vi "Funktionen Schalten NEU.vi"(8 "Fehler (Eingang)":errorcluster) -> (0 "Fehler (Ausgang)":errorcluster, 2 "Zustand":T1)   [LabVIEW 2020, in "Allgemein.lvlib"]
uses:
  Allgemein.lvlib
  Aktionen FGV Dichtheitstest.ctl
  Verwaltung/Verwaltung - cRIO.lvlib
  Verwaltung/FGV OUT Aktionen.ctl
  Regler/Regler.lvlib
  Regler/FGV Daten Regler Aktionen.ctl
  FGV Analysator aktiv.ctl
  Anlage Spuelen Aktionen.ctl
  FGV Zustaende Aktionen.ctl
  Aktion FGV Klima.ctl
  Funktionstasten/Zustaende.ctl
  Funktionstasten/Funktionstasten.lvlib
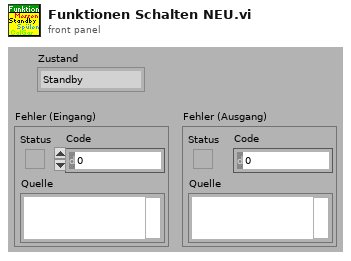
[diagram p1: front panel]
types:
  T1 = typedef "Funktionstasten.lvlib/Zustaende.ctl" = enum16{"Standby", "Pause", "Eco", "Messen", "Kalibrieren", "Spülen Filter", "Spülen Leitung", "Umgebungsluft", "0-Gas", "Cal-Gas", "CG zu PNS", "-------------", "Init 1", "Init 2", "Init 3", "Init 4", "Messen vorbereiten", "Messen durchführen", "Exit"}
  T2 = typedef "Allgemein.lvlib/Aktionen FGV Dichtheitstest.ctl" = enum16{"lesen", "schreiben"}
  T3 = typedef "Allgemein.lvlib/FGV Zustaende Aktionen.ctl" = enum16{"lesen", "Zustand PC", "Zustand cRIO", "Bildnummer", "Samplepoint", "Sysloglevel"}
  T4 = enum16{"Standby", "Pause", "Eco", "Messen", "Kalibrieren", "Spülen Filter", "Spülen Leitung", "Umgebungsluft", "0-Gas", "Cal-Gas 1", "CG zu PNS", "-------------", "Init 1", "Init 2", "Init 3", "Init 4", "Messen vorbereiten", "Messen durchführen", "Exit"}
  T5 = typedef "Regler.lvlib/FGV Daten Regler Aktionen.ctl" = enum16{"lesen", "Out%", "Heizung EIN"}
  T6 = typedef "Verwaltung - cRIO.lvlib/FGV OUT Aktionen.ctl" = enum16{"lesen", "ANA OUT", "DO 0-31", "DO 32-47"}
  T7 = typedef "Allgemein.lvlib/Anlage Spuelen Aktionen.ctl" = enum16{"lesen", "spülen?"}
  T8 = typedef "Allgemein.lvlib/FGV Analysator aktiv.ctl" = enum16{"lesen", "Analysator", "CG Aufschaltung", "KAL Zustand", "AutaKal GT?"}
  T9 = typedef "Allgemein.lvlib/Aktion FGV Klima.ctl" = enum16{"lesen", "Klimaanlage", "Container", "PNS"}
  T10 = typedef "EPA 1065.lvlib/Dichtheitstest 1065-345.lvlib/Aktion Leak check durchfuehren.ctl" = enum16{"initialisieren", "Unterdruck erzeugen", "Ventile schließen", "Warten", "Auswertung", "fertig", "PDF erstellen"}
  T11 = typedef "Erweiterte Konfig.lvlib/Aktionen Dichtheitstest.ctl" = enum16{"Initialisieren", "Unterdruck aufbauen", "Prop schließen", "Warten", "Auswertung", "Fertig"}
  T12 = cluster{"-20Y2":bool, "-20Y7":bool, "-21Y5":bool, "-22Y4":bool, "Absaugung":bool}
  T13 = typedef "Status Analysatoren.lvlib/Status Analysatoren_Anzeige.ctl" = cluster{"FT-IR":bool, "FID":bool, "PMA":bool}
  T14 = cluster{"20Y5":bool, "20Y6":bool, "20Y7":bool, "20Y8":bool, "21Y3":bool, "22Y3":bool, "23Y1":bool, "23Y2":bool, "23Y3":bool, "23Y4":bool, "27Y2":bool, "27Y3":bool, "27Y4":bool, "Absaugung":bool, "Kondensatpumpe":bool, "21Y5":bool}
  T15 = cluster{"-23Y1 (CG1)":bool, "-23Y2 (CG2)":bool, "-23Y3 (CG3-10)":bool, "-23Y4 (N2)":bool, "-23Y5":bool, "-27Y2":bool, "-20Y5":bool, "-20Y6":bool, "-20Y7":bool, "-20Y8":bool, "-27Y3":bool, "-27Y4":bool, "Pumpe":bool, "Kondensat":bool, "-22Y3":bool, "-20Y2":bool, "-21Y3":bool, "Absaugung":bool, "-21Y5":bool, "CG zu Entnahme":bool, "-20Y2 (CG3)":bool, "-20Y3 (CG4)":bool, "-20Y4 (CG5)":bool, "-20Y5 (CG6)":bool, "-20Y6 (CG7)":bool, "-20Y7 (CG8)":bool, "-20Y8 (CG9)":bool, "-21Y1 (CG10)":bool}
  T16 = typedef "Verwaltung - cRIO.lvlib/Digital Ausgaenge 32-63.ctl" = cluster{"O32: Messgaspumpe EIN":bool, "O33: (Umgebungsluftpumpe)":bool, "O34: (Kondensatpumpe GK)":bool, "O35: Klima/Lüfter EIN":bool, "O36: Versorgung Heizungen":bool, "O37: Versorgung Heizungen":bool, "O38: (Gaskühler EIN (Freigabe))":bool, "O39: Störung FAS LP":bool, "O40: (Heizung Filterblock)":bool, "O41: Heizung HL zu FT-IR":bool, "O42: Heizung HL Extern SP1":bool, "O43: Heizung HL Extern SP2":bool, "O44: Heizung Reserve":bool, "O45: Heizung Reserve":bool, "O46: Statusbeleuchtung grün":bool, "O47: Statusbeleuchtung rot":bool}
  T17 = typedef "Verwaltung - cRIO.lvlib/Digital Ausgaenge 0-31.ctl" = cluster{"O0: Druckluft Versorgung":bool, "O1: CG 3 (FB Eingang 1)":bool, "O2: CG 4 (Kühlung FT-IR EIN)":bool, "O3: CG 5 (FB Bypass)":bool, "O4: CG 6 (FB CalGas)":bool, "O5: CG 7 (FB spülen/UL)":bool, "O6: CG 8 (FB zum FT-IR)":bool, "O7: CG 9 (FB zum FID)":bool, "O8: CG 10 (FB Reserve)":bool, "O9: (FB Reserve)":bool, "O10: (FB Umgebungsluft FID)":bool, "O11: (FB zum Gaskühler)":bool, "O12: FB Stickstoff zu FT-IR":bool, "O13: (FB Druckluft/UL)":bool, "O14: (Purifier deaktivieren)":bool, "O15: (Umschaltung Purifier/Stickstoff)":bool, "O16: N2 Einblasung":bool, "O17: LSP LN2 Nachfüllung":bool, "O18: (Reserve)":bool, "O19: (Pumpe Eingang1)":bool, "O20: (Pumpe Eingang2)":bool, "O21: (Pumpe Spülen1)":bool, "O22: (Pumpe Spülen2)":bool, "O23: (Reserve)":bool, "O24: CalGas 1":bool, "O25: CalGas 2":bool, "O26: CG 3-10 (CalGas 3)":bool, "O27: Stickstoff aufschalten":bool, "O28: CG zu PNS":bool, "O29: FTIR Standby Spülung":bool, "O30: CG zu Entnahme(T90)":bool, "O31: (Purifier regenerieren)":bool}
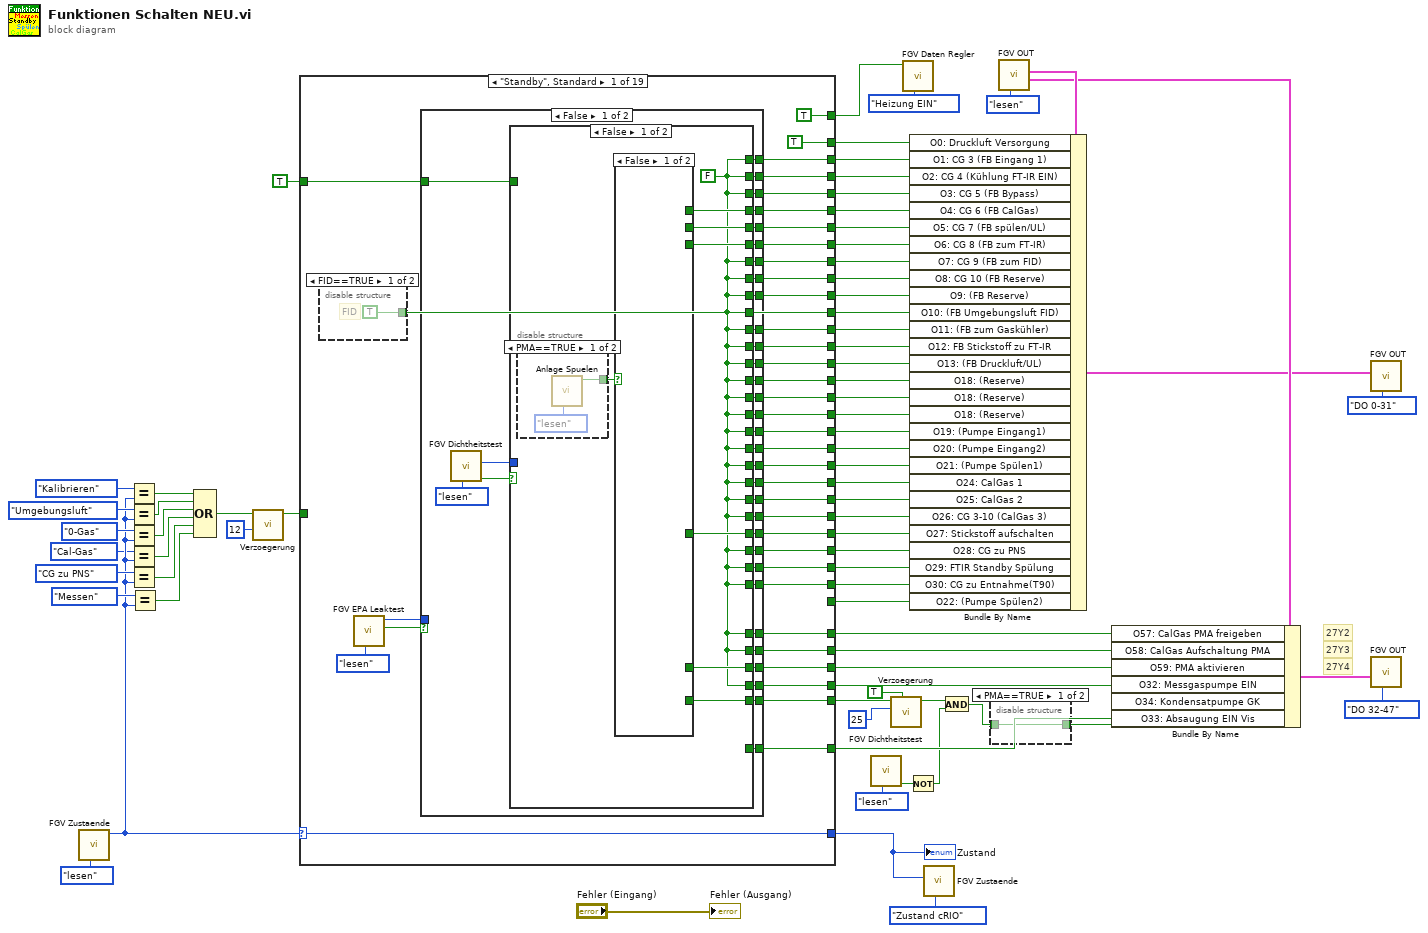
[diagram p0: block diagram]
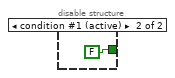
[diagram p2: hidden frame]
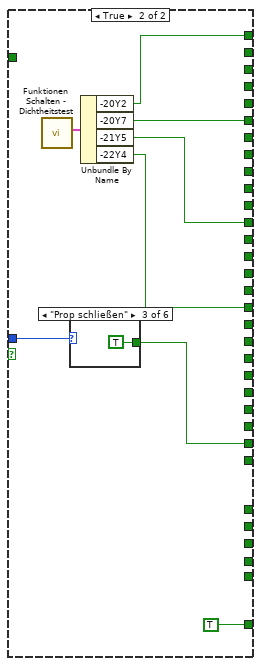
[diagram p6: hidden frame]
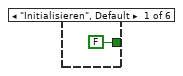
[diagram p7: hidden frame]
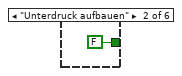
[diagram p8: hidden frame]
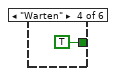
[diagram p9: hidden frame]
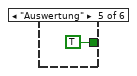
[diagram p10: hidden frame]
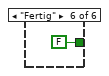
[diagram p11: hidden frame]
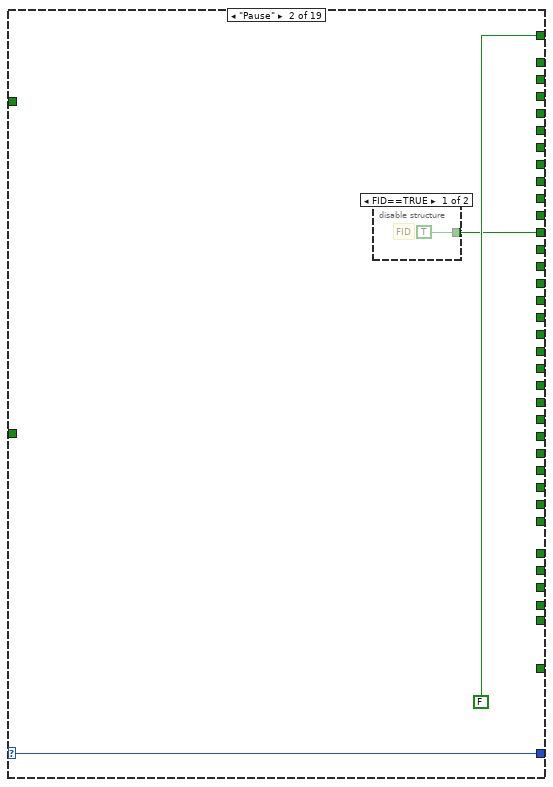
[diagram p18: hidden frame]
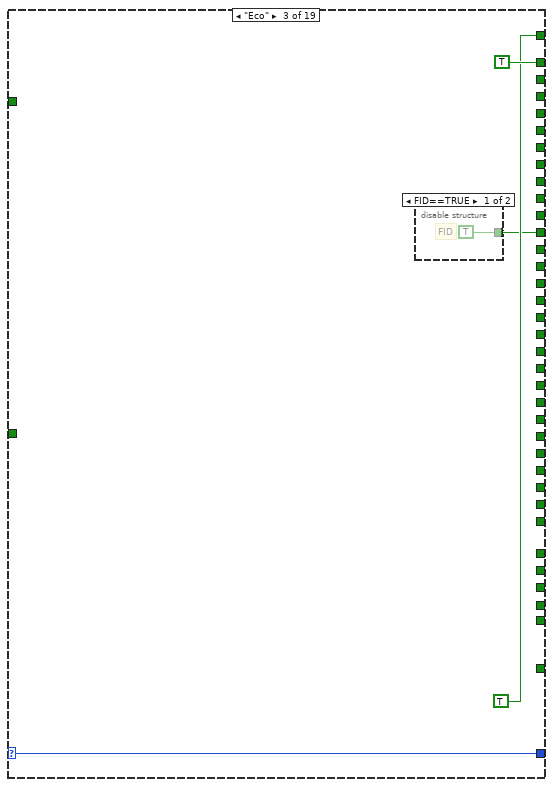
[diagram p20: hidden frame]
diagram:
  # "27Y4"
  # "27Y3"
  # "27Y2"
  n1 = call "FGV Zustaende.vi"("Aktionen"=FGV_Zustaende_Aktionen."lesen") -> ("Zustand PC"=w15:T1)  [unwired: 6 in, 4 out]
  n2 = Equal?(x=T4."Kalibrieren" ("Zustand PC"), y=w15) -> (x = y?=w37:bool)
  n3 = Equal?(x=T4."Umgebungsluft" ("Zustand PC"), y=w15) -> (x = y?=w36:bool)
  n4 = Equal?(x=T4."0-Gas" ("Zustand PC"), y=w15) -> (x = y?=w35:bool)
  n5 = Equal?(x=Zustaende."Cal-Gas", y=w15) -> (x = y?=w34:bool)
  n6 = Equal?(x=T4."CG zu PNS" ("Zustand PC"), y=w15) -> (x = y?=w33:bool)
  n7 = Equal?(x=T4."Messen" ("Zustand PC"), y=w15) -> (x = y?=w14:bool)
  n8 = Compound Arithmetic op=OR(w37, w36, w35, w34, w33, w14) -> (w31:bool)
  n9 = call "Verzoegerung.vi"("sec"=u16 12, "Startsignal"=w31) -> ("Zeit abgelaufen?"=w30:bool)  [unwired: 8 in, 1 out]
  n10 = case shown="\"Standby\", Standard" w15 {
    selector: w15 -> [w111 w181 w186 w206 w252 w328 w342 _ w371 w401 w423 _ _ _ _ _ _ _ _]
    tunnel: [w111 w181 w186 w206 w252 w328 w342 _ w371 w401 w423 _ _ _ _ _ _ _ _] -> w12
    tunnel: [w109 _ _ w191 w244 _ _ _ _ w397 w420 _ _ _ _ _ _ _ _] -> w72
    tunnel: [w108 _ _ _ _ _ _ _ _ _ _ _ _ _ _ _ _ _ _] -> w71
    tunnel: [w106 _ _ _ w247 _ _ _ w359 w396 w419 _ _ _ _ _ _ _ _] -> w68
    tunnel: [w105 _ _ w194 w239 w323 _ w356 w358 w395 w418 _ _ _ _ _ _ _ _] -> w67
    tunnel: [w104 _ _ w191 w243 _ _ w356 w359 w394 w417 _ _ _ _ _ _ _ _] -> w66
    tunnel: [w103 _ _ w200 w231 _ _ _ w365 w393 w416 _ _ _ _ _ _ _ _] -> w65
    tunnel: [w102 _ _ _ _ _ _ _ _ _ _ _ _ _ _ _ _ _ _] -> w61
    tunnel: [w82 w179 w183 w192 w232 w324 w336 _ w360 w392 w415 _ _ _ _ _ _ _ _] -> w60
    tunnel: [w83 _ _ w191 w245 w323 _ w356 w359 w382 w403 _ _ _ _ _ _ _ _] -> w59
    tunnel: [w101 _ _ _ _ w323 _ _ _ _ _ _ _ _ _ _ _ _ _] -> w56
    tunnel: TRUE -> [w110 _ _ w191 w248 w322 w339 w356 w359 _ _ _ _ _ _ _ _ _ _]
    tunnel: [w107 _ _ _ _ w325 _ _ _ _ _ _ _ _ _ _ _ _ _] -> w69
    tunnel: [w100 _ _ _ _ _ _ _ _ _ _ _ _ _ _ _ _ _ _] -> w57
    tunnel: [w92 _ _ w190 w240 _ _ _ w363 w376 w405 _ _ _ _ _ _ _ _] -> w24
    tunnel: [w93 _ _ w191 _ _ _ _ _ w384 w406 _ _ _ _ _ _ _ _] -> w64
    tunnel: [w95 _ _ _ w238 _ _ _ _ w391 w414 _ _ _ _ _ _ _ _] -> w50
    tunnel: [w96 _ _ _ _ _ w338 _ _ _ _ _ _ _ _ _ _ _ _] -> w53
    tunnel: [w97 _ _ w189 _ _ _ _ _ _ _ _ _ _ _ _ _ _ _] -> w52
    tunnel: [w98 _ _ w188 w227 _ _ _ _ _ _ _ _ _ _ _ _ _ _] -> w51
    tunnel: [w99 _ _ _ _ _ _ _ _ _ _ _ _ _ _ _ _ _ _] -> w54
    tunnel: [w94 _ _ _ w236 _ _ _ _ w389 w412 _ _ _ _ _ _ _ _] -> w49
    tunnel: [TRUE ("O0: Druckluft Versorgung") _ TRUE ("O0: Druckluft Versorgung") TRUE ("O0: Druckluft Versorgung") TRUE ("O0: Druckluft Versorgung") TRUE ("O0: Druckluft Versorgung") TRUE ("O0: Druckluft Versorgung") w357 TRUE ("O0: Druckluft Versorgung") TRUE ("O0: Druckluft Versorgung") TRUE ("O0: Druckluft Versorgung") TRUE ("O0: Druckluft Versorgung") TRUE ("O0: Druckluft Versorgung") TRUE ("O0: Druckluft Versorgung") TRUE ("O0: Druckluft Versorgung") TRUE ("O0: Druckluft Versorgung") TRUE ("O0: Druckluft Versorgung") TRUE ("O0: Druckluft Versorgung") TRUE ("O0: Druckluft Versorgung")] -> w63
    tunnel: [w90 _ _ _ _ _ _ _ _ _ _ _ _ _ _ _ _ _ _] -> w62
    tunnel: [w89 _ _ _ _ _ _ _ _ _ _ _ _ _ _ _ _ _ _] -> w58
    tunnel: [w88 _ _ _ _ _ _ _ _ _ _ _ _ _ _ _ _ _ _] -> w55
    tunnel: [w87 _ _ _ w237 _ _ _ _ w390 w413 _ _ _ _ _ _ _ _] -> w48
    tunnel: [w86 _ _ _ _ _ _ _ _ w387 w410 _ _ _ _ _ _ _ _] -> w47
    tunnel: [w85 _ _ _ w246 _ _ _ w359 w388 w411 _ _ _ _ _ _ _ _] -> w46
    tunnel: [TRUE ("Heizung AUS") FALSE ("Heizung AUS") TRUE ("Heizung AUS") TRUE ("Heizung AUS") TRUE ("Heizung AUS") TRUE ("Heizung AUS") TRUE ("Heizung AUS") w357 TRUE ("Heizung AUS") TRUE ("Heizung AUS") TRUE ("Heizung AUS") TRUE ("Heizung AUS") FALSE ("Heizung AUS") _ _ _ TRUE ("Heizung AUS") TRUE ("Heizung AUS") TRUE ("Heizung AUS")] -> w38
    tunnel: w30 -> [_ _ _ w201 w230 _ _ _ w364 _ _ _ _ _ _ _ _ _ _]
    tunnel: [w79 _ _ _ w235 _ _ _ _ w386 w409 _ _ _ _ _ _ _ _] -> w29
    tunnel: [w80 _ _ _ w234 _ _ _ _ w385 w408 _ _ _ _ _ _ _ _] -> w28
    tunnel: [w81 _ _ w195 w233 _ _ _ w363 w378 w407 _ _ _ _ _ _ _ _] -> w27
    tunnel: [w78 _ _ TRUE ("Absaugung") w241 _ _ w356 TRUE ("Absaugung") w383 w404 _ _ _ _ _ _ _ _] -> w22
    tunnel: [w76 _ _ _ w228 _ _ _ _ _ _ _ _ _ _ _ _ _ _] -> w11
    tunnel: [w77 _ _ _ _ _ _ _ _ _ _ _ _ _ _ _ _ _ _] -> w10
    tunnel: [_ _ _ _ _ _ w337 _ _ _ _ _ _ _ _ _ _ _ _] -> w1
    frame "Standby", Default {
      n11 = disable-structure shown="FID==TRUE" {
        disable-tunnel: [TRUE _] -> w82
        frame condition #0 {
          # "FID"
        }
        frame condition #1 (active) {
        }
      }
      n12 = call "FGV EPA Leaktest.vi"("Aktion"=enum16{"lesen", "schreiben"}."lesen") -> ("Leaktest aktiv"=w74:bool, "Leaktest Zustand"=w73:T10)  [unwired: 9 in]
      n13 = case shown="False" w74 {
        tunnel: w110 -> [w147 w173]
        tunnel: [w146 w173] -> w109
        tunnel: [w145 _] -> w108
        tunnel: [w144 _] -> w107
        tunnel: [w143 _] -> w106
        tunnel: [w142 _] -> w105
        tunnel: [w141 w173] -> w104
        tunnel: [w140 _] -> w103
        tunnel: [w139 _] -> w102
        tunnel: [w138 _] -> w101
        tunnel: [w137 _] -> w100
        tunnel: [w136 _] -> w99
        tunnel: [w135 w173] -> w98
        tunnel: [w134 _] -> w97
        tunnel: [w133 _] -> w96
        tunnel: [w132 _] -> w95
        tunnel: [w131 _] -> w94
        tunnel: [w130 _] -> w93
        tunnel: [w129 _] -> w92
        tunnel: [w126 _] -> w90
        tunnel: [w125 _] -> w89
        tunnel: [w124 _] -> w88
        tunnel: [w123 _] -> w87
        tunnel: [w122 _] -> w86
        tunnel: [w121 _] -> w85
        tunnel: [w120 w173] -> w83
        tunnel: [w119 _] -> w81
        tunnel: [w118 _] -> w80
        tunnel: [w117 _] -> w79
        tunnel: [w116 _] -> w78
        tunnel: [w114 _] -> w77
        tunnel: [w113 w175] -> w76
        tunnel: w73 -> [_ w174]
        frame False {
          n14 = call "FGV Dichtheitstest.vi"("Aktionen"=Aktionen_FGV_Dichtheitstest."lesen") -> ("Dichtheitstest?"=w127:bool, "Aktionen Dichtheitstest"=w115:T11)  [unwired: 9 in]
          n15 = case shown="False" w127 {
            tunnel: [w148 w165] -> w146
            tunnel: [w151 _] -> w129
            tunnel: [w148 _] -> w130
            tunnel: [w148 _] -> w131
            tunnel: [w148 _] -> w132
            tunnel: [w148 _] -> w133
            tunnel: [w148 _] -> w134
            tunnel: [w148 w159] -> w135
            tunnel: [w148 _] -> w136
            tunnel: [w148 _] -> w137
            tunnel: [w148 _] -> w138
            tunnel: [w148 _] -> _
            tunnel: [w148 _] -> w139
            tunnel: [w148 _] -> w140
            tunnel: [w149 w164] -> w141
            tunnel: [w152 _] -> w142
            tunnel: [w153 _] -> w143
            tunnel: [w148 _] -> w144
            tunnel: [w148 _] -> w145
            tunnel: w147 -> [_ _]
            tunnel: [w148 _] -> w126
            tunnel: [w148 _] -> w125
            tunnel: [w148 _] -> w124
            tunnel: [w148 _] -> w123
            tunnel: [w148 _] -> w122
            tunnel: [w154 _] -> w121
            tunnel: [w148 w163] -> w120
            tunnel: [w150 _] -> w119
            tunnel: [w148 _] -> w118
            tunnel: [w148 _] -> w117
            tunnel: [_ TRUE] -> w116
            tunnel: w115 -> [_ w161]
            tunnel: [w148 _] -> w114
            tunnel: [w148 w160] -> w113
            frame False {
              w148 = FALSE
              n16 = disable-structure shown="PMA==TRUE" {
                disable-tunnel: [w157 _] -> w155
                frame condition #0 {
                  n17 = call "Anlage Spuelen.vi"("Aktionen"=Anlage_Spuelen_Aktionen."lesen") -> ("Spülen?"=w157:bool)  [unwired: 10 in]
                }
                frame condition #1 (active) {
                }
              }
              n18 = case shown="False" w155 {
                selector: w155 -> [_ w158]
                tunnel: [_ w158] -> w154
                tunnel: [_ w158] -> w153
                tunnel: [_ w158] -> w152
                tunnel: [_ w158] -> w150
                tunnel: [_ w158] -> w151
                tunnel: [_ w158] -> w149
                frame False {
                }
                frame True {
                }
              }
            }
            frame True {
              n19 = call "Funktionen Schalten - Dichtheitstest.vi"() -> ("Ventile Dichtheitstest"=w166:T12)  [unwired: 11 in]
              n20 = case shown="\"Prop schließen\"" w161 {
                tunnel: [FALSE FALSE TRUE TRUE TRUE FALSE] -> w160
                frame "Initialisieren", Default {
                }
                frame "Unterdruck aufbauen" {
                }
                frame "Prop schließen" {
                }
                frame "Warten" {
                }
                frame "Auswertung" {
                }
                frame "Fertig" {
                }
              }
              n21 = Unbundle By Name(w166) -> ("-20Y2"=w165:bool, "-20Y7"=w164:bool, "-21Y5"=w163:bool, "-22Y4"=w159:bool)
            }
          }
        }
        frame True {
          n22 = case shown="\"Unterdruck erzeugen\"" w174 {
            tunnel: w173 -> [_ _ w176 w177 w178 _]
            tunnel: [_ _ w176 w177 w178 _] -> w175
            frame "initialisieren", Default {
            }
            frame "Unterdruck erzeugen" {
            }
            frame "Ventile schließen" {
            }
            frame "Warten" {
            }
            frame "Auswertung" {
            }
            frame "fertig" {
            }
          }
        }
      }
    }
    frame "Pause" {
      n23 = disable-structure shown="FID==TRUE" {
        disable-tunnel: [TRUE _] -> w179
        frame condition #0 {
          # "FID"
        }
        frame condition #1 (active) {
        }
      }
    }
    frame "Eco" {
      n24 = disable-structure shown="FID==TRUE" {
        disable-tunnel: [TRUE _] -> w183
        frame condition #0 {
          # "FID"
        }
        frame condition #1 (active) {
        }
      }
    }
    frame "Messen" {
      n25 = disable-structure shown="Deaktiviert" {
        disable-tunnel: [w208 _] -> w189
        disable-tunnel: [w207 _] -> w188
        frame Disabled {
          n26 = call "FGV Klima Option.vi"("Aktion"=Aktion_FGV_Klima."lesen") -> ("PNS vorhanden"=w209:bool)  [unwired: 8 in, 2 out]
          n27 = case shown="False" w209 {
            tunnel: [w212 FALSE] -> w208
            tunnel: [w211 TRUE] -> w207
            frame False {
              n28 = call "FGV Zustaende.vi"("Aktionen"=FGV_Zustaende_Aktionen."lesen") -> ("Samplepoint"=w213:u16)  [unwired: 6 in, 4 out]
              n29 = case shown="2" w213 {
                tunnel: [FALSE TRUE] -> w212
                tunnel: [TRUE FALSE] -> w211
                frame 1, Default {
                }
                frame 2 {
                }
              }
            }
            frame True {
            }
          }
        }
        frame Enabled {
        }
      }
      n30 = call "Anlage Spuelen.vi"("Aktionen"=Anlage_Spuelen_Aktionen."spülen?", "Spülen?"=TRUE) -> ()  [unwired: 9 in, 1 out]
      n31 = call "Analysator aktiv.vi"("Aktion"=FGV_Analysator_aktiv."lesen") -> ("Status Analysatoren"=w203:T13)  [unwired: 7 in, 3 out]
      n32 = Unbundle By Name(w203) -> ("FID"=w202:bool, "PMA"=w195:bool)
      n33 = And(x=w201, y=w202) -> (x .and. y?=w200:bool)
      n34 = disable-structure shown="PMA==TRUE" {
        disable-tunnel: [TRUE ("Spülen?") FALSE ("Spülen?")] -> w190
        frame condition #0 {
        }
        frame condition #1 (active) {
        }
      }
      n35 = disable-structure shown="PMA==TRUE" {
        disable-tunnel: [TRUE ("Spülen?") FALSE ("Spülen?")] -> w194
        frame condition #0 {
        }
        frame condition #1 (active) {
        }
      }
      n36 = Not(x=w200) -> (.not. x?=w193:bool)
      n37 = disable-structure shown="FID==TRUE" {
        disable-tunnel: w193 -> [w223 _]
        disable-tunnel: [w223 FALSE] -> w192
        frame condition #0 {
        }
        frame condition #1 (active) {
        }
      }
    }
    frame "Kalibrieren" {
      n38 = call "FGV Dichtheitstest.vi"("Aktionen"=Aktionen_FGV_Dichtheitstest."lesen") -> ("Dichtheitstest?"=w249:bool, "Aktionen Dichtheitstest"=w229:T11)  [unwired: 9 in]
      n39 = case shown="False" w249 {
        tunnel: w248 -> [_ _]
        tunnel: [w270 _] -> w247
        tunnel: [w260 TRUE] -> w241
        tunnel: [w264 _] -> w246
        tunnel: [w256 w312] -> w245
        tunnel: [w255 w313] -> w244
        tunnel: [w268 w311] -> w243
        tunnel: [w259 _] -> w240
        tunnel: [w269 _] -> w239
        tunnel: [w258 _] -> w231
        tunnel: [w267 _] -> w238
        tunnel: [w266 _] -> w237
        tunnel: [w265 _] -> w236
        tunnel: [w263 _] -> w235
        tunnel: [w262 _] -> w234
        tunnel: [w261 _] -> w233
        tunnel: w230 -> [w257 _]
        tunnel: w229 -> [_ w310]
        tunnel: [_ w309] -> w228
        tunnel: [_ w308] -> w227
        frame False {
          n40 = call "Analysator aktiv.vi"("Aktion"=FGV_Analysator_aktiv."lesen") -> ("Autokal GT?"=w253:u16)  [unwired: 7 in, 3 out]
          n41 = case shown="0, Standard" w253 {
            tunnel: [w287 w301] -> w270
            tunnel: [w286 w300] -> w269
            tunnel: [w285 w299] -> w268
            tunnel: [w283 w296] -> w267
            tunnel: [w282 w295] -> w266
            tunnel: [w281 w294] -> w265
            tunnel: [w280 w293] -> w264
            tunnel: [w274 w292] -> w263
            tunnel: [w279 w291] -> w262
            tunnel: [w278 w288] -> w261
            tunnel: [TRUE ("Kondensat") w289] -> w260
            tunnel: [TRUE ("Kondensat") w290] -> w259
            tunnel: [w277 w298] -> w258
            tunnel: w257 -> [w276 _]
            tunnel: [w275 w297] -> w256
            tunnel: [_ w302] -> w255
            frame 0, Default {
              n42 = call "Funktionen Schalten AutoKal.vi"() -> ("AutoKal"=w271:T14)  [unwired: 11 in]
              n43 = Unbundle By Name(w271) -> ("20Y5"=w287:bool, "20Y6"=w286:bool, "20Y7"=w285:bool, "20Y8"=w284:bool, "21Y5"=w275:bool, "23Y1"=w283:bool, "23Y2"=w282:bool, "23Y3"=w281:bool, "23Y4"=w280:bool, "27Y2"=w274:bool, "27Y3"=w279:bool, "27Y4"=w278:bool)  [unwired: 1 out]
              n44 = And(x=w284, y=w276) -> (x .and. y?=w277:bool)
            }
            frame 1 {
              n45 = call "CalGas aufschalten.vi"() -> ("Cluster"=w307:T15)  [unwired: 11 in]
              n46 = call "Analysator aktiv.vi"("Aktion"=FGV_Analysator_aktiv."lesen") -> ("Status Analysatoren"=w306:T13)  [unwired: 7 in, 3 out]
              n47 = Unbundle By Name(w307) -> ("-20Y2"=w302:bool, "-20Y5"=w301:bool, "-20Y6"=w300:bool, "-20Y7"=w299:bool, "-20Y8"=w298:bool, "-21Y5"=w297:bool, "-23Y1 (CG1)"=w296:bool, "-23Y2 (CG2)"=w295:bool, "-23Y3 (CG3-10)"=w294:bool, "-23Y4 (N2)"=w293:bool, "-27Y2"=w292:bool, "-27Y3"=w291:bool, "-27Y4"=w304:bool, "Kondensat"=w290:bool, "Absaugung"=w289:bool)  [unwired: 3 out]
              n48 = Unbundle By Name(w306) -> ("PMA"=w303:bool)
              n49 = And(x=w304, y=w303) -> (x .and. y?=w288:bool)
            }
          }
        }
        frame True {
          n50 = call "Funktionen Schalten - Dichtheitstest.vi"() -> ("Ventile Dichtheitstest"=w314:T12)  [unwired: 11 in]
          n51 = Unbundle By Name(w314) -> ("-20Y2"=w313:bool, "-20Y7"=w311:bool, "-21Y5"=w312:bool, "-22Y4"=w308:bool)
          n52 = case shown="\"Fertig\"" w310 {
            tunnel: [FALSE FALSE TRUE TRUE TRUE FALSE] -> w309
            frame "Initialisieren", Default {
            }
            frame "Unterdruck aufbauen" {
            }
            frame "Prop schließen" {
            }
            frame "Warten" {
            }
            frame "Auswertung" {
            }
            frame "Fertig" {
            }
          }
        }
      }
      n53 = Not(x=w231) -> (.not. x?=w232:bool)
    }
    frame "Spülen Filter" {
      n54 = disable-structure shown="Filter_Spuelen==FALSE, Standard" {
        disable-tunnel: [w330 w332] -> w325
        disable-tunnel: [w329 w332] -> w323
        disable-tunnel: w322 -> [w329 _]
        frame condition #0 {
          n55 = call "Taktmerker.vi"("Aktion"=enum16{"lesen", "bearbeiten"}."lesen") -> ("1 s"=w330:bool)  [unwired: 6 in, 4 out]
        }
        frame condition #1 (active) {
          w332 = FALSE
        }
      }
      n56 = disable-structure shown="FID==TRUE" {
        disable-tunnel: [TRUE _] -> w324
        frame condition #0 {
          # "FID"
        }
        frame condition #1 (active) {
        }
      }
    }
    frame "Spülen Leitung" {
      n57 = call "FGV Klima Option.vi"("Aktion"=Aktion_FGV_Klima."lesen") -> ("PNS vorhanden"=w334:bool)  [unwired: 8 in, 2 out]
      n58 = disable-structure shown="Pumpe_Spuelen==FALSE, Standard" {
        disable-tunnel: w339 -> [w347 _]
        disable-tunnel: [w346 w355] -> w338
        disable-tunnel: [w345 w355] -> w337
        disable-tunnel: w334 -> [w344 _]
        frame condition #0 {
          n59 = case shown="False" w344 {
            tunnel: w347 -> [w352 _]
            tunnel: [w351 _] -> w346
            tunnel: [w350 _] -> w345
            frame False {
              n60 = call "FGV Zustaende.vi"("Aktionen"=FGV_Zustaende_Aktionen."lesen") -> ("Samplepoint"=w348:u16)  [unwired: 6 in, 4 out]
              n61 = case shown="1, Standard" w348 {
                tunnel: w352 -> [w353 w354]
                tunnel: [w353 _] -> w351
                tunnel: [_ w354] -> w350
                frame 1, Default {
                }
                frame 2 {
                }
              }
            }
            frame True {
            }
          }
        }
        frame condition #1 (active) {
          w355 = FALSE
        }
      }
      n62 = disable-structure shown="FID==TRUE" {
        disable-tunnel: [TRUE _] -> w336
        frame condition #0 {
          # "FID"
        }
        frame condition #1 (active) {
        }
      }
    }
    frame "Umgebungsluft" {
      w357 = TRUE
    }
    frame "0-Gas" {
      n63 = call "Analysator aktiv.vi"("Aktion"=FGV_Analysator_aktiv."lesen") -> ("Status Analysatoren"=w367:T13)  [unwired: 7 in, 3 out]
      n64 = Unbundle By Name(w367) -> ("FID"=w366:bool, "PMA"=w363:bool)
      n65 = And(x=w364, y=w366) -> (x .and. y?=w365:bool)
      n66 = Not(x=w365) -> (.not. x?=w361:bool)
      n67 = disable-structure shown="PMA==TRUE" {
        disable-tunnel: [TRUE ("Spülen?") FALSE ("Spülen?")] -> w358
        frame condition #0 {
        }
        frame condition #1 (active) {
        }
      }
      n68 = disable-structure shown="FID==TRUE" {
        disable-tunnel: w361 -> [w374 _]
        disable-tunnel: [w374 FALSE] -> w360
        frame condition #0 {
        }
        frame condition #1 (active) {
        }
      }
    }
    frame "Cal-Gas" {
      n69 = call "CalGas aufschalten.vi"() -> ("Cluster"=w399:T15)  [unwired: 11 in]
      n70 = Unbundle By Name(w399) -> ("-20Y2"=w397:bool, "-20Y5"=w396:bool, "-20Y6"=w395:bool, "-20Y7"=w394:bool, "-20Y8"=w393:bool, "-21Y3"=w392:bool, "-21Y5"=w382:bool, "-23Y1 (CG1)"=w391:bool, "-23Y2 (CG2)"=w390:bool, "-23Y3 (CG3-10)"=w389:bool, "-23Y4 (N2)"=w388:bool, "-23Y5"=w387:bool, "-27Y2"=w386:bool, "-27Y3"=w385:bool, "-27Y4"=w379:bool, "Pumpe"=w384:bool, "Kondensat"=w376:bool, "Absaugung"=w383:bool)
      n71 = call "Analysator aktiv.vi"("Aktion"=FGV_Analysator_aktiv."lesen") -> ("Status Analysatoren"=w381:T13)  [unwired: 7 in, 3 out]
      n72 = Unbundle By Name(w381) -> ("PMA"=w377:bool)
      n73 = And(x=w379, y=w377) -> (x .and. y?=w378:bool)
    }
    frame "CG zu PNS" {
      n74 = call "CalGas aufschalten.vi"() -> ("Cluster"=w402:T15)  [unwired: 11 in]
      n75 = Unbundle By Name(w402) -> ("-20Y2"=w420:bool, "-20Y5"=w419:bool, "-20Y6"=w418:bool, "-20Y7"=w417:bool, "-20Y8"=w416:bool, "-21Y3"=w415:bool, "-21Y5"=w403:bool, "-23Y1 (CG1)"=w414:bool, "-23Y2 (CG2)"=w413:bool, "-23Y3 (CG3-10)"=w412:bool, "-23Y4 (N2)"=w411:bool, "-23Y5"=w410:bool, "-27Y2"=w409:bool, "-27Y3"=w408:bool, "-27Y4"=w407:bool, "Pumpe"=w406:bool, "Kondensat"=w405:bool, "Absaugung"=w404:bool)
    }
    frame "-------------" {
    }
    frame "Init 1" {
    }
    frame "Init 2" {
    }
    frame "Init 3" {
    }
    frame "Init 4" {
    }
    frame "Messen vorbereiten" {
    }
    frame "Messen durchführen" {
    }
    frame "Exit" {
    }
  }
  "Zustand" <- w12
  n76 = call "FGV Dichtheitstest.vi"("Aktionen"=Aktionen_FGV_Dichtheitstest."lesen") -> ("Dichtheitstest?"=w6:bool)  [unwired: 9 in, 1 out]
  n77 = call "Verzoegerung.vi"("Abfallverzögerung?"=TRUE, "min"=u16 25 ("sec"), "Startsignal"=w24) -> ("Zeit abgelaufen?"=w7:bool)  [unwired: 7 in, 1 out]
  n78 = call "FGV Daten Regler.vi"("Aktionen"=FGV_Daten_Regler_Aktionen."Heizung EIN", "Heizung EIN"=w38) -> ()  [unwired: 8 in, 2 out]
  n79 = Not(x=w6) -> (.not. x?=w5:bool)
  n80 = call "FGV Zustaende.vi"("Aktionen"=FGV_Zustaende_Aktionen."Zustand cRIO", "Zustand cRIO"=w12) -> ()  [unwired: 5 in, 5 out]
  n81 = And(x=w7, y=w5) -> (x .and. y?=w3:bool)
  n82 = disable-structure shown="PMA==TRUE" {
    disable-tunnel: [w437 FALSE ("Spülen?")] -> w2
    disable-tunnel: w3 -> [w437 _]
    frame condition #0 {
    }
    frame condition #1 (active) {
    }
  }
  n83 = call "FGV OUT.vi"("Aktion"=FGV_OUT_Aktionen."lesen") -> ("DO 32-63"=w43:T16, "DO 0-31"=w44:T17)  [unwired: 7 in, 2 out]
  n84 = Bundle By Name(cluster=w44, "O0: Druckluft Versorgung"=w63, "O1: CG 3 (FB Eingang 1)"=w72, "O2: CG 4 (Kühlung FT-IR EIN)"=w71, "O3: CG 5 (FB Bypass)"=w69, "O4: CG 6 (FB CalGas)"=w68, "O5: CG 7 (FB spülen/UL)"=w67, "O6: CG 8 (FB zum FT-IR)"=w66, "O7: CG 9 (FB zum FID)"=w65, "O8: CG 10 (FB Reserve)"=w62, "O9: (FB Reserve)"=w61, "O10: (FB Umgebungsluft FID)"=w60, "O11: (FB zum Gaskühler)"=w58, "O12: FB Stickstoff zu FT-IR"=w59, "O13: (FB Druckluft/UL)"=w56, "O18: (Reserve)"=w57, "O18: (Reserve)"=w55, "O18: (Reserve)"=w54, "O19: (Pumpe Eingang1)"=w51, "O20: (Pumpe Eingang2)"=w52, "O21: (Pumpe Spülen1)"=w53, "O24: CalGas 1"=w50, "O25: CalGas 2"=w48, "O26: CG 3-10 (CalGas 3)"=w49, "O27: Stickstoff aufschalten"=w46, "O28: CG zu PNS"=w47, "O29: FTIR Standby Spülung"=w11, "O30: CG zu Entnahme(T90)"=w10, "O22: (Pumpe Spülen2)"=w1) -> (w23:T17)
  n85 = Bundle By Name(cluster=w43, "O57: CalGas PMA freigeben"=w29, "O58: CalGas Aufschaltung PMA"=w28, "O59: PMA aktivieren"=w27, "O32: Messgaspumpe EIN"=w64, "O34: Kondensatpumpe GK"=w2, "O33: Absaugung EIN Vis"=w22) -> (w40:T16)
  n86 = call "FGV OUT.vi"("Aktion"=FGV_OUT_Aktionen."DO 0-31", "DO 0-31"=w23) -> ()  [unwired: 6 in, 4 out]
  n87 = call "FGV OUT.vi"("Aktion"=FGV_OUT_Aktionen."DO 32-47", "DO 32-63"=w40) -> ()  [unwired: 6 in, 4 out]
  "Fehler (Ausgang)" <- "Fehler (Eingang)"
